vi "update waveform plot names.vi"(10 "selected plot names":string[](array[string]), 11 "WaveformChart in":refnum<vi>) -> ()   [LabVIEW 2016]
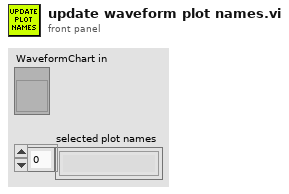
[diagram p1: front panel]
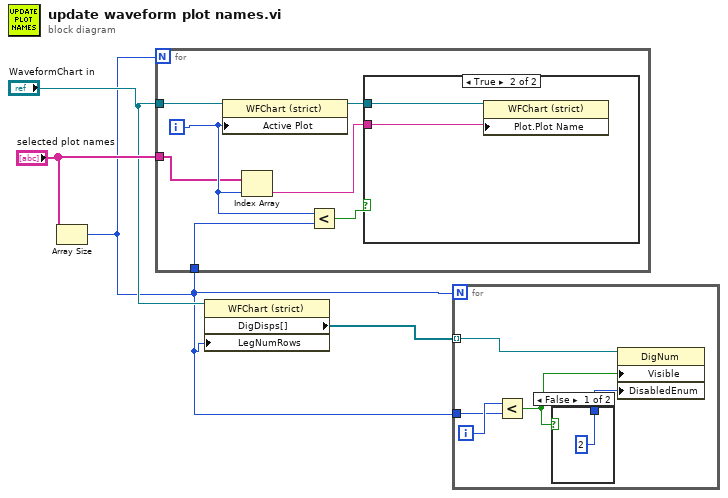
[diagram p0: block diagram]
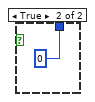
[diagram p2: hidden frame]
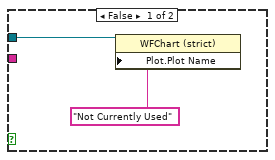
[diagram p3: hidden frame]
diagram:
  n1 = Array Size(array="selected plot names") -> (size(s)=w1:i32)
  n2 = for {
    N: w1 -> [_]
    tunnel: "WaveformChart in" -> [w11]
    tunnel: "selected plot names" -> [w6]
    tunnel: w1 -> [w9]
    i -> [w7]
    n3 = property class="WFChart (strict)"(reference=w11, "Active Plot"=w7) -> (reference out=w10:refnum<vi>)  [unwired: 1 in, 1 out]
    n4 = Index Array(array=w6, index=w7) -> (element=w5:string)
    n5 = Less?(x=w7, y=w9) -> (x < y?=w8:bool)
    n6 = case shown="True" w8 {
      tunnel: w10 -> [w13 w15]
      tunnel: w5 -> [_ w14]
      frame False {
        n7 = property class="WFChart (strict)"(reference=w13, "Plot.Plot Name"="Not Currently Used") -> ()  [unwired: 1 in, 2 out]
      }
      frame True {
        n8 = property class="WFChart (strict)"(reference=w15, "Plot.Plot Name"=w14) -> ()  [unwired: 1 in, 2 out]
      }
    }
  }
  n9 = property class="WFChart (strict)"(reference="WaveformChart in", "LegNumRows"=w1) -> ("DigDisps[]"=w3:refnum<vi>[])  [unwired: 1 in, 2 out]
  n10 = for {
    N: w1 -> [_]
    tunnel: w3 -> [w20] mode=indexing
    tunnel: w1 -> [w18]
    i -> [w19]
    n11 = Less?(x=w19, y=w18) -> (x < y?=w17:bool)
    n12 = case shown="False" w17 {
      tunnel: [2 0] -> w16
      frame False {
      }
      frame True {
      }
    }
    n13 = property class="DigNum"(reference=w20, "Visible"=w17, "DisabledEnum"=w16) -> ()  [unwired: 1 in, 2 out]
  }
